vi "数字量输出配置.vi"() -> ()   [LabVIEW 2010] (continued)
              n3559 = local write "单选_第72路"(w107) -> ()
              n3560 = local write "单选_第73路"(w107) -> ()
              n3561 = local write "单选_第74路"(w107) -> ()
              n3562 = local write "单选_第75路"(w107) -> ()
              n3563 = local write "单选_第76路"(w107) -> ()
              n3564 = local write "单选_第77路"(w107) -> ()
              n3565 = local write "单选_第78路"(w107) -> ()
              n3566 = local write "单选_第80路"(w107) -> ()
            }
            frame 40 {
              w108 = TRUE
              w109 = FALSE ("单选_第41路")
              n3567 = local write "单选_第1路"(w108) -> ()
              n3568 = local write "单选_第2路"(w108) -> ()
              n3569 = local write "单选_第3路"(w108) -> ()
              n3570 = local write "单选_第4路"(w108) -> ()
              n3571 = local write "单选_第5路"(w108) -> ()
              n3572 = local write "单选_第6路"(w108) -> ()
              n3573 = local write "单选_第7路"(w108) -> ()
              n3574 = local write "单选_第8路"(w108) -> ()
              n3575 = local write "单选_第9路"(w108) -> ()
              n3576 = local write "单选_第10路"(w108) -> ()
              n3577 = local write "单选_第11路"(w108) -> ()
              n3578 = local write "单选_第12路"(w108) -> ()
              n3579 = local write "单选_第13路"(w108) -> ()
              n3580 = local write "单选_第14路"(w108) -> ()
              n3581 = local write "单选_第15路"(w108) -> ()
              n3582 = local write "单选_第16路"(w108) -> ()
              n3583 = local write "单选_第17路"(w108) -> ()
              n3584 = local write "单选_第18路"(w108) -> ()
              n3585 = local write "单选_第19路"(w108) -> ()
              n3586 = local write "单选_第20路"(w108) -> ()
              n3587 = local write "单选_第21路"(w108) -> ()
              n3588 = local write "单选_第22路"(w108) -> ()
              n3589 = local write "单选_第23路"(w108) -> ()
              n3590 = local write "单选_第24路"(w108) -> ()
              n3591 = local write "单选_第25路"(w108) -> ()
              n3592 = local write "单选_第26路"(w108) -> ()
              n3593 = local write "单选_第27路"(w108) -> ()
              n3594 = local write "单选_第28路"(w108) -> ()
              n3595 = local write "单选_第29路"(w108) -> ()
              n3596 = local write "单选_第30路"(w108) -> ()
              n3597 = local write "单选_第31路"(w108) -> ()
              n3598 = local write "单选_第32路"(w108) -> ()
              n3599 = local write "单选_第33路"(w108) -> ()
              n3600 = local write "单选_第34路"(w108) -> ()
              n3601 = local write "单选_第35路"(w108) -> ()
              n3602 = local write "单选_第36路"(w108) -> ()
              n3603 = local write "单选_第37路"(w108) -> ()
              n3604 = local write "单选_第38路"(w108) -> ()
              n3605 = local write "单选_第39路"(w108) -> ()
              n3606 = local write "单选_第40路"(w108) -> ()
              n3607 = local write "单选_第41路"(w109) -> ()
              n3608 = local write "单选_第42路"(w109) -> ()
              n3609 = local write "单选_第43路"(w109) -> ()
              n3610 = local write "单选_第44路"(w109) -> ()
              n3611 = local write "单选_第45路"(w109) -> ()
              n3612 = local write "单选_第46路"(w109) -> ()
              n3613 = local write "单选_第47路"(w109) -> ()
              n3614 = local write "单选_第48路"(w109) -> ()
              n3615 = local write "单选_第49路"(w109) -> ()
              n3616 = local write "单选_第50路"(w109) -> ()
              n3617 = local write "单选_第51路"(w109) -> ()
              n3618 = local write "单选_第52路"(w109) -> ()
              n3619 = local write "单选_第53路"(w109) -> ()
              n3620 = local write "单选_第54路"(w109) -> ()
              n3621 = local write "单选_第55路"(w109) -> ()
              n3622 = local write "单选_第56路"(w109) -> ()
              n3623 = local write "单选_第57路"(w109) -> ()
              n3624 = local write "单选_第58路"(w109) -> ()
              n3625 = local write "单选_第59路"(w109) -> ()
              n3626 = local write "单选_第60路"(w109) -> ()
              n3627 = local write "单选_第61路"(w109) -> ()
              n3628 = local write "单选_第62路"(w109) -> ()
              n3629 = local write "单选_第63路"(w109) -> ()
              n3630 = local write "单选_第64路"(w109) -> ()
              n3631 = local write "单选_第71路"(w109) -> ()
              n3632 = local write "单选_第79路"(w109) -> ()
              n3633 = local write "单选_第65路"(w109) -> ()
              n3634 = local write "单选_第66路"(w109) -> ()
              n3635 = local write "单选_第67路"(w109) -> ()
              n3636 = local write "单选_第68路"(w109) -> ()
              n3637 = local write "单选_第69路"(w109) -> ()
              n3638 = local write "单选_第70路"(w109) -> ()
              n3639 = local write "单选_第72路"(w109) -> ()
              n3640 = local write "单选_第73路"(w109) -> ()
              n3641 = local write "单选_第74路"(w109) -> ()
              n3642 = local write "单选_第75路"(w109) -> ()
              n3643 = local write "单选_第76路"(w109) -> ()
              n3644 = local write "单选_第77路"(w109) -> ()
              n3645 = local write "单选_第78路"(w109) -> ()
              n3646 = local write "单选_第80路"(w109) -> ()
            }
            frame 41 {
              w110 = TRUE
              w111 = FALSE ("单选_第41路")
              n3647 = local write "单选_第1路"(w110) -> ()
              n3648 = local write "单选_第2路"(w110) -> ()
              n3649 = local write "单选_第3路"(w110) -> ()
              n3650 = local write "单选_第4路"(w110) -> ()
              n3651 = local write "单选_第5路"(w110) -> ()
              n3652 = local write "单选_第6路"(w110) -> ()
              n3653 = local write "单选_第7路"(w110) -> ()
              n3654 = local write "单选_第8路"(w110) -> ()
              n3655 = local write "单选_第9路"(w110) -> ()
              n3656 = local write "单选_第10路"(w110) -> ()
              n3657 = local write "单选_第11路"(w110) -> ()
              n3658 = local write "单选_第12路"(w110) -> ()
              n3659 = local write "单选_第13路"(w110) -> ()
              n3660 = local write "单选_第14路"(w110) -> ()
              n3661 = local write "单选_第15路"(w110) -> ()
              n3662 = local write "单选_第16路"(w110) -> ()
              n3663 = local write "单选_第17路"(w110) -> ()
              n3664 = local write "单选_第18路"(w110) -> ()
              n3665 = local write "单选_第19路"(w110) -> ()
              n3666 = local write "单选_第20路"(w110) -> ()
              n3667 = local write "单选_第21路"(w110) -> ()
              n3668 = local write "单选_第22路"(w110) -> ()
              n3669 = local write "单选_第23路"(w110) -> ()
              n3670 = local write "单选_第24路"(w110) -> ()
              n3671 = local write "单选_第25路"(w110) -> ()
              n3672 = local write "单选_第26路"(w110) -> ()
              n3673 = local write "单选_第27路"(w110) -> ()
              n3674 = local write "单选_第28路"(w110) -> ()
              n3675 = local write "单选_第29路"(w110) -> ()
              n3676 = local write "单选_第30路"(w110) -> ()
              n3677 = local write "单选_第31路"(w110) -> ()
              n3678 = local write "单选_第32路"(w110) -> ()
              n3679 = local write "单选_第33路"(w110) -> ()
              n3680 = local write "单选_第34路"(w110) -> ()
              n3681 = local write "单选_第35路"(w110) -> ()
              n3682 = local write "单选_第36路"(w110) -> ()
              n3683 = local write "单选_第37路"(w110) -> ()
              n3684 = local write "单选_第38路"(w110) -> ()
              n3685 = local write "单选_第39路"(w110) -> ()
              n3686 = local write "单选_第40路"(w110) -> ()
              n3687 = local write "单选_第41路"(w110) -> ()
              n3688 = local write "单选_第42路"(w111) -> ()
              n3689 = local write "单选_第43路"(w111) -> ()
              n3690 = local write "单选_第44路"(w111) -> ()
              n3691 = local write "单选_第45路"(w111) -> ()
              n3692 = local write "单选_第46路"(w111) -> ()
              n3693 = local write "单选_第47路"(w111) -> ()
              n3694 = local write "单选_第48路"(w111) -> ()
              n3695 = local write "单选_第49路"(w111) -> ()
              n3696 = local write "单选_第50路"(w111) -> ()
              n3697 = local write "单选_第51路"(w111) -> ()
              n3698 = local write "单选_第52路"(w111) -> ()
              n3699 = local write "单选_第53路"(w111) -> ()
              n3700 = local write "单选_第54路"(w111) -> ()
              n3701 = local write "单选_第55路"(w111) -> ()
              n3702 = local write "单选_第56路"(w111) -> ()
              n3703 = local write "单选_第57路"(w111) -> ()
              n3704 = local write "单选_第58路"(w111) -> ()
              n3705 = local write "单选_第59路"(w111) -> ()
              n3706 = local write "单选_第60路"(w111) -> ()
              n3707 = local write "单选_第61路"(w111) -> ()
              n3708 = local write "单选_第62路"(w111) -> ()
              n3709 = local write "单选_第63路"(w111) -> ()
              n3710 = local write "单选_第64路"(w111) -> ()
              n3711 = local write "单选_第71路"(w111) -> ()
              n3712 = local write "单选_第79路"(w111) -> ()
              n3713 = local write "单选_第65路"(w111) -> ()
              n3714 = local write "单选_第66路"(w111) -> ()
              n3715 = local write "单选_第67路"(w111) -> ()
              n3716 = local write "单选_第68路"(w111) -> ()
              n3717 = local write "单选_第69路"(w111) -> ()
              n3718 = local write "单选_第70路"(w111) -> ()
              n3719 = local write "单选_第72路"(w111) -> ()
              n3720 = local write "单选_第73路"(w111) -> ()
              n3721 = local write "单选_第74路"(w111) -> ()
              n3722 = local write "单选_第75路"(w111) -> ()
              n3723 = local write "单选_第76路"(w111) -> ()
              n3724 = local write "单选_第77路"(w111) -> ()
              n3725 = local write "单选_第78路"(w111) -> ()
              n3726 = local write "单选_第80路"(w111) -> ()
            }
            frame 42 {
              w112 = TRUE
              w113 = FALSE ("单选_第41路")
              n3727 = local write "单选_第1路"(w112) -> ()
              n3728 = local write "单选_第2路"(w112) -> ()
              n3729 = local write "单选_第3路"(w112) -> ()
              n3730 = local write "单选_第4路"(w112) -> ()
              n3731 = local write "单选_第5路"(w112) -> ()
              n3732 = local write "单选_第6路"(w112) -> ()
              n3733 = local write "单选_第7路"(w112) -> ()
              n3734 = local write "单选_第8路"(w112) -> ()
              n3735 = local write "单选_第9路"(w112) -> ()
              n3736 = local write "单选_第10路"(w112) -> ()
              n3737 = local write "单选_第11路"(w112) -> ()
              n3738 = local write "单选_第12路"(w112) -> ()
              n3739 = local write "单选_第13路"(w112) -> ()
              n3740 = local write "单选_第14路"(w112) -> ()
              n3741 = local write "单选_第15路"(w112) -> ()
              n3742 = local write "单选_第16路"(w112) -> ()
              n3743 = local write "单选_第17路"(w112) -> ()
              n3744 = local write "单选_第18路"(w112) -> ()
              n3745 = local write "单选_第19路"(w112) -> ()
              n3746 = local write "单选_第20路"(w112) -> ()
              n3747 = local write "单选_第21路"(w112) -> ()
              n3748 = local write "单选_第22路"(w112) -> ()
              n3749 = local write "单选_第23路"(w112) -> ()
              n3750 = local write "单选_第24路"(w112) -> ()
              n3751 = local write "单选_第25路"(w112) -> ()
              n3752 = local write "单选_第26路"(w112) -> ()
              n3753 = local write "单选_第27路"(w112) -> ()
              n3754 = local write "单选_第28路"(w112) -> ()
              n3755 = local write "单选_第29路"(w112) -> ()
              n3756 = local write "单选_第30路"(w112) -> ()
              n3757 = local write "单选_第31路"(w112) -> ()
              n3758 = local write "单选_第32路"(w112) -> ()
              n3759 = local write "单选_第33路"(w112) -> ()
              n3760 = local write "单选_第34路"(w112) -> ()
              n3761 = local write "单选_第35路"(w112) -> ()
              n3762 = local write "单选_第36路"(w112) -> ()
              n3763 = local write "单选_第37路"(w112) -> ()
              n3764 = local write "单选_第38路"(w112) -> ()
              n3765 = local write "单选_第39路"(w112) -> ()
              n3766 = local write "单选_第40路"(w112) -> ()
              n3767 = local write "单选_第41路"(w112) -> ()
              n3768 = local write "单选_第42路"(w112) -> ()
              n3769 = local write "单选_第43路"(w113) -> ()
              n3770 = local write "单选_第44路"(w113) -> ()
              n3771 = local write "单选_第45路"(w113) -> ()
              n3772 = local write "单选_第46路"(w113) -> ()
              n3773 = local write "单选_第47路"(w113) -> ()
              n3774 = local write "单选_第48路"(w113) -> ()
              n3775 = local write "单选_第49路"(w113) -> ()
              n3776 = local write "单选_第50路"(w113) -> ()
              n3777 = local write "单选_第51路"(w113) -> ()
              n3778 = local write "单选_第52路"(w113) -> ()
              n3779 = local write "单选_第53路"(w113) -> ()
              n3780 = local write "单选_第54路"(w113) -> ()
              n3781 = local write "单选_第55路"(w113) -> ()
              n3782 = local write "单选_第56路"(w113) -> ()
              n3783 = local write "单选_第57路"(w113) -> ()
              n3784 = local write "单选_第58路"(w113) -> ()
              n3785 = local write "单选_第59路"(w113) -> ()
              n3786 = local write "单选_第60路"(w113) -> ()
              n3787 = local write "单选_第61路"(w113) -> ()
              n3788 = local write "单选_第62路"(w113) -> ()
              n3789 = local write "单选_第63路"(w113) -> ()
              n3790 = local write "单选_第64路"(w113) -> ()
              n3791 = local write "单选_第71路"(w113) -> ()
              n3792 = local write "单选_第79路"(w113) -> ()
              n3793 = local write "单选_第65路"(w113) -> ()
              n3794 = local write "单选_第66路"(w113) -> ()
              n3795 = local write "单选_第67路"(w113) -> ()
              n3796 = local write "单选_第68路"(w113) -> ()
              n3797 = local write "单选_第69路"(w113) -> ()
              n3798 = local write "单选_第70路"(w113) -> ()
              n3799 = local write "单选_第72路"(w113) -> ()
              n3800 = local write "单选_第73路"(w113) -> ()
              n3801 = local write "单选_第74路"(w113) -> ()
              n3802 = local write "单选_第75路"(w113) -> ()
              n3803 = local write "单选_第76路"(w113) -> ()
              n3804 = local write "单选_第77路"(w113) -> ()
              n3805 = local write "单选_第78路"(w113) -> ()
              n3806 = local write "单选_第80路"(w113) -> ()
            }
            frame 43 {
              w114 = TRUE
              w115 = FALSE ("单选_第41路")
              n3807 = local write "单选_第1路"(w114) -> ()
              n3808 = local write "单选_第2路"(w114) -> ()
              n3809 = local write "单选_第3路"(w114) -> ()
              n3810 = local write "单选_第4路"(w114) -> ()
              n3811 = local write "单选_第5路"(w114) -> ()
              n3812 = local write "单选_第6路"(w114) -> ()
              n3813 = local write "单选_第7路"(w114) -> ()
              n3814 = local write "单选_第8路"(w114) -> ()
              n3815 = local write "单选_第9路"(w114) -> ()
              n3816 = local write "单选_第10路"(w114) -> ()
              n3817 = local write "单选_第11路"(w114) -> ()
              n3818 = local write "单选_第12路"(w114) -> ()
              n3819 = local write "单选_第13路"(w114) -> ()
              n3820 = local write "单选_第14路"(w114) -> ()
              n3821 = local write "单选_第15路"(w114) -> ()
              n3822 = local write "单选_第16路"(w114) -> ()
              n3823 = local write "单选_第17路"(w114) -> ()
              n3824 = local write "单选_第18路"(w114) -> ()
              n3825 = local write "单选_第19路"(w114) -> ()
              n3826 = local write "单选_第20路"(w114) -> ()
              n3827 = local write "单选_第21路"(w114) -> ()
              n3828 = local write "单选_第22路"(w114) -> ()
              n3829 = local write "单选_第23路"(w114) -> ()
              n3830 = local write "单选_第24路"(w114) -> ()
              n3831 = local write "单选_第25路"(w114) -> ()
              n3832 = local write "单选_第26路"(w114) -> ()
              n3833 = local write "单选_第27路"(w114) -> ()
              n3834 = local write "单选_第28路"(w114) -> ()
              n3835 = local write "单选_第29路"(w114) -> ()
              n3836 = local write "单选_第30路"(w114) -> ()
              n3837 = local write "单选_第31路"(w114) -> ()
              n3838 = local write "单选_第32路"(w114) -> ()
              n3839 = local write "单选_第33路"(w114) -> ()
              n3840 = local write "单选_第34路"(w114) -> ()
              n3841 = local write "单选_第35路"(w114) -> ()
              n3842 = local write "单选_第36路"(w114) -> ()
              n3843 = local write "单选_第37路"(w114) -> ()
              n3844 = local write "单选_第38路"(w114) -> ()
              n3845 = local write "单选_第39路"(w114) -> ()
              n3846 = local write "单选_第40路"(w114) -> ()
              n3847 = local write "单选_第41路"(w114) -> ()
              n3848 = local write "单选_第42路"(w114) -> ()
              n3849 = local write "单选_第43路"(w114) -> ()
              n3850 = local write "单选_第44路"(w115) -> ()
              n3851 = local write "单选_第45路"(w115) -> ()
              n3852 = local write "单选_第46路"(w115) -> ()
              n3853 = local write "单选_第47路"(w115) -> ()
              n3854 = local write "单选_第48路"(w115) -> ()
              n3855 = local write "单选_第49路"(w115) -> ()
              n3856 = local write "单选_第50路"(w115) -> ()
              n3857 = local write "单选_第51路"(w115) -> ()
              n3858 = local write "单选_第52路"(w115) -> ()
              n3859 = local write "单选_第53路"(w115) -> ()
              n3860 = local write "单选_第54路"(w115) -> ()
              n3861 = local write "单选_第55路"(w115) -> ()
              n3862 = local write "单选_第56路"(w115) -> ()
              n3863 = local write "单选_第57路"(w115) -> ()
              n3864 = local write "单选_第58路"(w115) -> ()
              n3865 = local write "单选_第59路"(w115) -> ()
              n3866 = local write "单选_第60路"(w115) -> ()
              n3867 = local write "单选_第61路"(w115) -> ()
              n3868 = local write "单选_第62路"(w115) -> ()
              n3869 = local write "单选_第63路"(w115) -> ()
              n3870 = local write "单选_第64路"(w115) -> ()
              n3871 = local write "单选_第71路"(w115) -> ()
              n3872 = local write "单选_第79路"(w115) -> ()
              n3873 = local write "单选_第65路"(w115) -> ()
              n3874 = local write "单选_第66路"(w115) -> ()
              n3875 = local write "单选_第67路"(w115) -> ()
              n3876 = local write "单选_第68路"(w115) -> ()
              n3877 = local write "单选_第69路"(w115) -> ()
              n3878 = local write "单选_第70路"(w115) -> ()
              n3879 = local write "单选_第72路"(w115) -> ()
              n3880 = local write "单选_第73路"(w115) -> ()
              n3881 = local write "单选_第74路"(w115) -> ()
              n3882 = local write "单选_第75路"(w115) -> ()
              n3883 = local write "单选_第76路"(w115) -> ()
              n3884 = local write "单选_第77路"(w115) -> ()
              n3885 = local write "单选_第78路"(w115) -> ()
              n3886 = local write "单选_第80路"(w115) -> ()
            }
            frame 44 {
              w116 = TRUE
              w117 = FALSE ("单选_第41路")
              n3887 = local write "单选_第1路"(w116) -> ()
              n3888 = local write "单选_第2路"(w116) -> ()
              n3889 = local write "单选_第3路"(w116) -> ()
              n3890 = local write "单选_第4路"(w116) -> ()
              n3891 = local write "单选_第5路"(w116) -> ()
              n3892 = local write "单选_第6路"(w116) -> ()
              n3893 = local write "单选_第7路"(w116) -> ()
              n3894 = local write "单选_第8路"(w116) -> ()
              n3895 = local write "单选_第9路"(w116) -> ()
              n3896 = local write "单选_第10路"(w116) -> ()
              n3897 = local write "单选_第11路"(w116) -> ()
              n3898 = local write "单选_第12路"(w116) -> ()
              n3899 = local write "单选_第13路"(w116) -> ()
              n3900 = local write "单选_第14路"(w116) -> ()
              n3901 = local write "单选_第15路"(w116) -> ()
              n3902 = local write "单选_第16路"(w116) -> ()
              n3903 = local write "单选_第17路"(w116) -> ()
              n3904 = local write "单选_第18路"(w116) -> ()
              n3905 = local write "单选_第19路"(w116) -> ()
              n3906 = local write "单选_第20路"(w116) -> ()
              n3907 = local write "单选_第21路"(w116) -> ()
              n3908 = local write "单选_第22路"(w116) -> ()
              n3909 = local write "单选_第23路"(w116) -> ()
              n3910 = local write "单选_第24路"(w116) -> ()
              n3911 = local write "单选_第25路"(w116) -> ()
              n3912 = local write "单选_第26路"(w116) -> ()
              n3913 = local write "单选_第27路"(w116) -> ()
              n3914 = local write "单选_第28路"(w116) -> ()
              n3915 = local write "单选_第29路"(w116) -> ()
              n3916 = local write "单选_第30路"(w116) -> ()
              n3917 = local write "单选_第31路"(w116) -> ()
              n3918 = local write "单选_第32路"(w116) -> ()
              n3919 = local write "单选_第33路"(w116) -> ()
              n3920 = local write "单选_第34路"(w116) -> ()
              n3921 = local write "单选_第35路"(w116) -> ()
              n3922 = local write "单选_第36路"(w116) -> ()
              n3923 = local write "单选_第37路"(w116) -> ()
              n3924 = local write "单选_第38路"(w116) -> ()
              n3925 = local write "单选_第39路"(w116) -> ()
              n3926 = local write "单选_第40路"(w116) -> ()
              n3927 = local write "单选_第41路"(w116) -> ()
              n3928 = local write "单选_第42路"(w116) -> ()
              n3929 = local write "单选_第43路"(w116) -> ()
              n3930 = local write "单选_第44路"(w116) -> ()
              n3931 = local write "单选_第45路"(w117) -> ()
              n3932 = local write "单选_第46路"(w117) -> ()
              n3933 = local write "单选_第47路"(w117) -> ()
              n3934 = local write "单选_第48路"(w117) -> ()
              n3935 = local write "单选_第49路"(w117) -> ()
              n3936 = local write "单选_第50路"(w117) -> ()
              n3937 = local write "单选_第51路"(w117) -> ()
              n3938 = local write "单选_第52路"(w117) -> ()
              n3939 = local write "单选_第53路"(w117) -> ()
              n3940 = local write "单选_第54路"(w117) -> ()
              n3941 = local write "单选_第55路"(w117) -> ()
              n3942 = local write "单选_第56路"(w117) -> ()
              n3943 = local write "单选_第57路"(w117) -> ()
              n3944 = local write "单选_第58路"(w117) -> ()
              n3945 = local write "单选_第59路"(w117) -> ()
              n3946 = local write "单选_第60路"(w117) -> ()
              n3947 = local write "单选_第61路"(w117) -> ()
              n3948 = local write "单选_第62路"(w117) -> ()
              n3949 = local write "单选_第63路"(w117) -> ()
              n3950 = local write "单选_第64路"(w117) -> ()
              n3951 = local write "单选_第71路"(w117) -> ()
              n3952 = local write "单选_第79路"(w117) -> ()
              n3953 = local write "单选_第65路"(w117) -> ()
              n3954 = local write "单选_第66路"(w117) -> ()
              n3955 = local write "单选_第67路"(w117) -> ()
              n3956 = local write "单选_第68路"(w117) -> ()
              n3957 = local write "单选_第69路"(w117) -> ()
              n3958 = local write "单选_第70路"(w117) -> ()
              n3959 = local write "单选_第72路"(w117) -> ()
              n3960 = local write "单选_第73路"(w117) -> ()
              n3961 = local write "单选_第74路"(w117) -> ()
              n3962 = local write "单选_第75路"(w117) -> ()
              n3963 = local write "单选_第76路"(w117) -> ()
              n3964 = local write "单选_第77路"(w117) -> ()
              n3965 = local write "单选_第78路"(w117) -> ()
              n3966 = local write "单选_第80路"(w117) -> ()
            }
            frame 45 {
              w118 = TRUE
              w119 = FALSE ("单选_第41路")
              n3967 = local write "单选_第1路"(w118) -> ()
              n3968 = local write "单选_第2路"(w118) -> ()
              n3969 = local write "单选_第3路"(w118) -> ()
              n3970 = local write "单选_第4路"(w118) -> ()
              n3971 = local write "单选_第5路"(w118) -> ()
              n3972 = local write "单选_第6路"(w118) -> ()
              n3973 = local write "单选_第7路"(w118) -> ()
              n3974 = local write "单选_第8路"(w118) -> ()
              n3975 = local write "单选_第9路"(w118) -> ()
              n3976 = local write "单选_第10路"(w118) -> ()
              n3977 = local write "单选_第11路"(w118) -> ()
              n3978 = local write "单选_第12路"(w118) -> ()
              n3979 = local write "单选_第13路"(w118) -> ()
              n3980 = local write "单选_第14路"(w118) -> ()
              n3981 = local write "单选_第15路"(w118) -> ()
              n3982 = local write "单选_第16路"(w118) -> ()
              n3983 = local write "单选_第17路"(w118) -> ()
              n3984 = local write "单选_第18路"(w118) -> ()
              n3985 = local write "单选_第19路"(w118) -> ()
              n3986 = local write "单选_第20路"(w118) -> ()
              n3987 = local write "单选_第21路"(w118) -> ()
              n3988 = local write "单选_第22路"(w118) -> ()
              n3989 = local write "单选_第23路"(w118) -> ()
              n3990 = local write "单选_第24路"(w118) -> ()
              n3991 = local write "单选_第25路"(w118) -> ()
              n3992 = local write "单选_第26路"(w118) -> ()
              n3993 = local write "单选_第27路"(w118) -> ()
              n3994 = local write "单选_第28路"(w118) -> ()
              n3995 = local write "单选_第29路"(w118) -> ()
              n3996 = local write "单选_第30路"(w118) -> ()
              n3997 = local write "单选_第31路"(w118) -> ()
              n3998 = local write "单选_第32路"(w118) -> ()
              n3999 = local write "单选_第33路"(w118) -> ()
              n4000 = local write "单选_第34路"(w118) -> ()
              n4001 = local write "单选_第35路"(w118) -> ()
              n4002 = local write "单选_第36路"(w118) -> ()
              n4003 = local write "单选_第37路"(w118) -> ()
              n4004 = local write "单选_第38路"(w118) -> ()
              n4005 = local write "单选_第39路"(w118) -> ()
              n4006 = local write "单选_第40路"(w118) -> ()
              n4007 = local write "单选_第41路"(w118) -> ()
              n4008 = local write "单选_第42路"(w118) -> ()
              n4009 = local write "单选_第43路"(w118) -> ()
              n4010 = local write "单选_第44路"(w118) -> ()
              n4011 = local write "单选_第45路"(w118) -> ()
              n4012 = local write "单选_第46路"(w119) -> ()
              n4013 = local write "单选_第47路"(w119) -> ()
              n4014 = local write "单选_第48路"(w119) -> ()
              n4015 = local write "单选_第49路"(w119) -> ()
              n4016 = local write "单选_第50路"(w119) -> ()
              n4017 = local write "单选_第51路"(w119) -> ()
              n4018 = local write "单选_第52路"(w119) -> ()
              n4019 = local write "单选_第53路"(w119) -> ()
              n4020 = local write "单选_第54路"(w119) -> ()
              n4021 = local write "单选_第55路"(w119) -> ()
              n4022 = local write "单选_第56路"(w119) -> ()
              n4023 = local write "单选_第57路"(w119) -> ()
              n4024 = local write "单选_第58路"(w119) -> ()
              n4025 = local write "单选_第59路"(w119) -> ()
              n4026 = local write "单选_第60路"(w119) -> ()
              n4027 = local write "单选_第61路"(w119) -> ()
              n4028 = local write "单选_第62路"(w119) -> ()
              n4029 = local write "单选_第63路"(w119) -> ()
              n4030 = local write "单选_第64路"(w119) -> ()
              n4031 = local write "单选_第71路"(w119) -> ()
              n4032 = local write "单选_第79路"(w119) -> ()
              n4033 = local write "单选_第65路"(w119) -> ()
              n4034 = local write "单选_第66路"(w119) -> ()
              n4035 = local write "单选_第67路"(w119) -> ()
              n4036 = local write "单选_第68路"(w119) -> ()
              n4037 = local write "单选_第69路"(w119) -> ()
              n4038 = local write "单选_第70路"(w119) -> ()
              n4039 = local write "单选_第72路"(w119) -> ()
              n4040 = local write "单选_第73路"(w119) -> ()
              n4041 = local write "单选_第74路"(w119) -> ()
              n4042 = local write "单选_第75路"(w119) -> ()
              n4043 = local write "单选_第76路"(w119) -> ()
              n4044 = local write "单选_第77路"(w119) -> ()
              n4045 = local write "单选_第78路"(w119) -> ()
              n4046 = local write "单选_第80路"(w119) -> ()
            }
            frame 46 {
              w120 = TRUE
              w121 = FALSE ("单选_第41路")
              n4047 = local write "单选_第1路"(w120) -> ()
              n4048 = local write "单选_第2路"(w120) -> ()
              n4049 = local write "单选_第3路"(w120) -> ()
              n4050 = local write "单选_第4路"(w120) -> ()
              n4051 = local write "单选_第5路"(w120) -> ()
              n4052 = local write "单选_第6路"(w120) -> ()
              n4053 = local write "单选_第7路"(w120) -> ()
              n4054 = local write "单选_第8路"(w120) -> ()
              n4055 = local write "单选_第9路"(w120) -> ()
              n4056 = local write "单选_第10路"(w120) -> ()
              n4057 = local write "单选_第11路"(w120) -> ()
              n4058 = local write "单选_第12路"(w120) -> ()
              n4059 = local write "单选_第13路"(w120) -> ()
              n4060 = local write "单选_第14路"(w120) -> ()
              n4061 = local write "单选_第15路"(w120) -> ()
              n4062 = local write "单选_第16路"(w120) -> ()
              n4063 = local write "单选_第17路"(w120) -> ()
              n4064 = local write "单选_第18路"(w120) -> ()
              n4065 = local write "单选_第19路"(w120) -> ()
              n4066 = local write "单选_第20路"(w120) -> ()
              n4067 = local write "单选_第21路"(w120) -> ()
              n4068 = local write "单选_第22路"(w120) -> ()
              n4069 = local write "单选_第23路"(w120) -> ()
              n4070 = local write "单选_第24路"(w120) -> ()
              n4071 = local write "单选_第25路"(w120) -> ()
              n4072 = local write "单选_第26路"(w120) -> ()
              n4073 = local write "单选_第27路"(w120) -> ()
              n4074 = local write "单选_第28路"(w120) -> ()
              n4075 = local write "单选_第29路"(w120) -> ()
              n4076 = local write "单选_第30路"(w120) -> ()
              n4077 = local write "单选_第31路"(w120) -> ()
              n4078 = local write "单选_第32路"(w120) -> ()
              n4079 = local write "单选_第33路"(w120) -> ()
              n4080 = local write "单选_第34路"(w120) -> ()
              n4081 = local write "单选_第35路"(w120) -> ()
              n4082 = local write "单选_第36路"(w120) -> ()
              n4083 = local write "单选_第37路"(w120) -> ()
              n4084 = local write "单选_第38路"(w120) -> ()
              n4085 = local write "单选_第39路"(w120) -> ()
              n4086 = local write "单选_第40路"(w120) -> ()
              n4087 = local write "单选_第41路"(w120) -> ()
              n4088 = local write "单选_第42路"(w120) -> ()
              n4089 = local write "单选_第43路"(w120) -> ()
              n4090 = local write "单选_第44路"(w120) -> ()
              n4091 = local write "单选_第45路"(w120) -> ()
              n4092 = local write "单选_第46路"(w120) -> ()
              n4093 = local write "单选_第47路"(w121) -> ()
              n4094 = local write "单选_第48路"(w121) -> ()
              n4095 = local write "单选_第49路"(w121) -> ()
              n4096 = local write "单选_第50路"(w121) -> ()
              n4097 = local write "单选_第51路"(w121) -> ()
              n4098 = local write "单选_第52路"(w121) -> ()
              n4099 = local write "单选_第53路"(w121) -> ()
              n4100 = local write "单选_第54路"(w121) -> ()
              n4101 = local write "单选_第55路"(w121) -> ()
              n4102 = local write "单选_第56路"(w121) -> ()
              n4103 = local write "单选_第57路"(w121) -> ()
              n4104 = local write "单选_第58路"(w121) -> ()
              n4105 = local write "单选_第59路"(w121) -> ()
              n4106 = local write "单选_第60路"(w121) -> ()
              n4107 = local write "单选_第61路"(w121) -> ()
              n4108 = local write "单选_第62路"(w121) -> ()
              n4109 = local write "单选_第63路"(w121) -> ()
              n4110 = local write "单选_第64路"(w121) -> ()
              n4111 = local write "单选_第71路"(w121) -> ()
              n4112 = local write "单选_第79路"(w121) -> ()
              n4113 = local write "单选_第65路"(w121) -> ()
              n4114 = local write "单选_第66路"(w121) -> ()
              n4115 = local write "单选_第67路"(w121) -> ()
              n4116 = local write "单选_第68路"(w121) -> ()
              n4117 = local write "单选_第69路"(w121) -> ()
              n4118 = local write "单选_第70路"(w121) -> ()
              n4119 = local write "单选_第72路"(w121) -> ()
              n4120 = local write "单选_第73路"(w121) -> ()
              n4121 = local write "单选_第74路"(w121) -> ()
              n4122 = local write "单选_第75路"(w121) -> ()
              n4123 = local write "单选_第76路"(w121) -> ()
              n4124 = local write "单选_第77路"(w121) -> ()
              n4125 = local write "单选_第78路"(w121) -> ()
              n4126 = local write "单选_第80路"(w121) -> ()
            }
            frame 47 {
              w122 = TRUE
              w123 = FALSE ("单选_第41路")
              n4127 = local write "单选_第1路"(w122) -> ()
              n4128 = local write "单选_第2路"(w122) -> ()
              n4129 = local write "单选_第3路"(w122) -> ()
              n4130 = local write "单选_第4路"(w122) -> ()
              n4131 = local write "单选_第5路"(w122) -> ()
              n4132 = local write "单选_第6路"(w122) -> ()
              n4133 = local write "单选_第7路"(w122) -> ()
              n4134 = local write "单选_第8路"(w122) -> ()
              n4135 = local write "单选_第9路"(w122) -> ()
              n4136 = local write "单选_第10路"(w122) -> ()
              n4137 = local write "单选_第11路"(w122) -> ()
              n4138 = local write "单选_第12路"(w122) -> ()
              n4139 = local write "单选_第13路"(w122) -> ()
              n4140 = local write "单选_第14路"(w122) -> ()
              n4141 = local write "单选_第15路"(w122) -> ()
              n4142 = local write "单选_第16路"(w122) -> ()
              n4143 = local write "单选_第17路"(w122) -> ()
              n4144 = local write "单选_第18路"(w122) -> ()
              n4145 = local write "单选_第19路"(w122) -> ()
              n4146 = local write "单选_第20路"(w122) -> ()
              n4147 = local write "单选_第21路"(w122) -> ()
              n4148 = local write "单选_第22路"(w122) -> ()
              n4149 = local write "单选_第23路"(w122) -> ()
              n4150 = local write "单选_第24路"(w122) -> ()
              n4151 = local write "单选_第25路"(w122) -> ()
              n4152 = local write "单选_第26路"(w122) -> ()
              n4153 = local write "单选_第27路"(w122) -> ()
              n4154 = local write "单选_第28路"(w122) -> ()
              n4155 = local write "单选_第29路"(w122) -> ()
              n4156 = local write "单选_第30路"(w122) -> ()
              n4157 = local write "单选_第31路"(w122) -> ()
              n4158 = local write "单选_第32路"(w122) -> ()
              n4159 = local write "单选_第33路"(w122) -> ()
              n4160 = local write "单选_第34路"(w122) -> ()
              n4161 = local write "单选_第35路"(w122) -> ()
              n4162 = local write "单选_第36路"(w122) -> ()
              n4163 = local write "单选_第37路"(w122) -> ()
              n4164 = local write "单选_第38路"(w122) -> ()
              n4165 = local write "单选_第39路"(w122) -> ()
              n4166 = local write "单选_第40路"(w122) -> ()
              n4167 = local write "单选_第41路"(w122) -> ()
              n4168 = local write "单选_第42路"(w122) -> ()
              n4169 = local write "单选_第43路"(w122) -> ()
              n4170 = local write "单选_第44路"(w122) -> ()
              n4171 = local write "单选_第45路"(w122) -> ()
              n4172 = local write "单选_第46路"(w122) -> ()
              n4173 = local write "单选_第47路"(w122) -> ()
              n4174 = local write "单选_第48路"(w123) -> ()
              n4175 = local write "单选_第49路"(w123) -> ()
              n4176 = local write "单选_第50路"(w123) -> ()
              n4177 = local write "单选_第51路"(w123) -> ()
              n4178 = local write "单选_第52路"(w123) -> ()
              n4179 = local write "单选_第53路"(w123) -> ()
              n4180 = local write "单选_第54路"(w123) -> ()
              n4181 = local write "单选_第55路"(w123) -> ()
              n4182 = local write "单选_第56路"(w123) -> ()
              n4183 = local write "单选_第57路"(w123) -> ()
              n4184 = local write "单选_第58路"(w123) -> ()
              n4185 = local write "单选_第59路"(w123) -> ()
              n4186 = local write "单选_第60路"(w123) -> ()
              n4187 = local write "单选_第61路"(w123) -> ()
              n4188 = local write "单选_第62路"(w123) -> ()
              n4189 = local write "单选_第63路"(w123) -> ()
              n4190 = local write "单选_第64路"(w123) -> ()
              n4191 = local write "单选_第71路"(w123) -> ()
              n4192 = local write "单选_第79路"(w123) -> ()
              n4193 = local write "单选_第65路"(w123) -> ()
              n4194 = local write "单选_第66路"(w123) -> ()
              n4195 = local write "单选_第67路"(w123) -> ()
              n4196 = local write "单选_第68路"(w123) -> ()
              n4197 = local write "单选_第69路"(w123) -> ()
              n4198 = local write "单选_第70路"(w123) -> ()
              n4199 = local write "单选_第72路"(w123) -> ()
              n4200 = local write "单选_第73路"(w123) -> ()
              n4201 = local write "单选_第74路"(w123) -> ()
              n4202 = local write "单选_第75路"(w123) -> ()
              n4203 = local write "单选_第76路"(w123) -> ()
              n4204 = local write "单选_第77路"(w123) -> ()
              n4205 = local write "单选_第78路"(w123) -> ()
              n4206 = local write "单选_第80路"(w123) -> ()
            }
            frame 48 {
              w124 = TRUE
              w125 = FALSE ("单选_第41路")
              n4207 = local write "单选_第1路"(w124) -> ()
              n4208 = local write "单选_第2路"(w124) -> ()
              n4209 = local write "单选_第3路"(w124) -> ()
              n4210 = local write "单选_第4路"(w124) -> ()
              n4211 = local write "单选_第5路"(w124) -> ()
              n4212 = local write "单选_第6路"(w124) -> ()
              n4213 = local write "单选_第7路"(w124) -> ()
              n4214 = local write "单选_第8路"(w124) -> ()
              n4215 = local write "单选_第9路"(w124) -> ()
              n4216 = local write "单选_第10路"(w124) -> ()
              n4217 = local write "单选_第11路"(w124) -> ()
              n4218 = local write "单选_第12路"(w124) -> ()
              n4219 = local write "单选_第13路"(w124) -> ()
              n4220 = local write "单选_第14路"(w124) -> ()
              n4221 = local write "单选_第15路"(w124) -> ()
              n4222 = local write "单选_第16路"(w124) -> ()
              n4223 = local write "单选_第17路"(w124) -> ()
              n4224 = local write "单选_第18路"(w124) -> ()
              n4225 = local write "单选_第19路"(w124) -> ()
              n4226 = local write "单选_第20路"(w124) -> ()
              n4227 = local write "单选_第21路"(w124) -> ()
              n4228 = local write "单选_第22路"(w124) -> ()
              n4229 = local write "单选_第23路"(w124) -> ()
              n4230 = local write "单选_第24路"(w124) -> ()
              n4231 = local write "单选_第25路"(w124) -> ()
              n4232 = local write "单选_第26路"(w124) -> ()
              n4233 = local write "单选_第27路"(w124) -> ()
              n4234 = local write "单选_第28路"(w124) -> ()
              n4235 = local write "单选_第29路"(w124) -> ()
              n4236 = local write "单选_第30路"(w124) -> ()
              n4237 = local write "单选_第31路"(w124) -> ()
              n4238 = local write "单选_第32路"(w124) -> ()
              n4239 = local write "单选_第33路"(w124) -> ()
              n4240 = local write "单选_第34路"(w124) -> ()
              n4241 = local write "单选_第35路"(w124) -> ()
              n4242 = local write "单选_第36路"(w124) -> ()
              n4243 = local write "单选_第37路"(w124) -> ()
              n4244 = local write "单选_第38路"(w124) -> ()
              n4245 = local write "单选_第39路"(w124) -> ()
              n4246 = local write "单选_第40路"(w124) -> ()
              n4247 = local write "单选_第41路"(w124) -> ()
              n4248 = local write "单选_第42路"(w124) -> ()
              n4249 = local write "单选_第43路"(w124) -> ()
              n4250 = local write "单选_第44路"(w124) -> ()
              n4251 = local write "单选_第45路"(w124) -> ()
              n4252 = local write "单选_第46路"(w124) -> ()
              n4253 = local write "单选_第47路"(w124) -> ()
              n4254 = local write "单选_第48路"(w124) -> ()
              n4255 = local write "单选_第49路"(w125) -> ()
              n4256 = local write "单选_第50路"(w125) -> ()
              n4257 = local write "单选_第51路"(w125) -> ()
              n4258 = local write "单选_第52路"(w125) -> ()
              n4259 = local write "单选_第53路"(w125) -> ()
              n4260 = local write "单选_第54路"(w125) -> ()
              n4261 = local write "单选_第55路"(w125) -> ()
              n4262 = local write "单选_第56路"(w125) -> ()
              n4263 = local write "单选_第57路"(w125) -> ()
              n4264 = local write "单选_第58路"(w125) -> ()
              n4265 = local write "单选_第59路"(w125) -> ()
              n4266 = local write "单选_第60路"(w125) -> ()
              n4267 = local write "单选_第61路"(w125) -> ()
              n4268 = local write "单选_第62路"(w125) -> ()
              n4269 = local write "单选_第63路"(w125) -> ()
              n4270 = local write "单选_第64路"(w125) -> ()
              n4271 = local write "单选_第71路"(w125) -> ()
              n4272 = local write "单选_第79路"(w125) -> ()
              n4273 = local write "单选_第65路"(w125) -> ()
              n4274 = local write "单选_第66路"(w125) -> ()
              n4275 = local write "单选_第67路"(w125) -> ()
              n4276 = local write "单选_第68路"(w125) -> ()
              n4277 = local write "单选_第69路"(w125) -> ()
              n4278 = local write "单选_第70路"(w125) -> ()
              n4279 = local write "单选_第72路"(w125) -> ()
              n4280 = local write "单选_第73路"(w125) -> ()
              n4281 = local write "单选_第74路"(w125) -> ()
              n4282 = local write "单选_第75路"(w125) -> ()
              n4283 = local write "单选_第76路"(w125) -> ()
              n4284 = local write "单选_第77路"(w125) -> ()
              n4285 = local write "单选_第78路"(w125) -> ()
              n4286 = local write "单选_第80路"(w125) -> ()
            }
            frame 49 {
              w126 = TRUE
              w127 = FALSE ("单选_第41路")
              n4287 = local write "单选_第1路"(w126) -> ()
              n4288 = local write "单选_第2路"(w126) -> ()
              n4289 = local write "单选_第3路"(w126) -> ()
              n4290 = local write "单选_第4路"(w126) -> ()
              n4291 = local write "单选_第5路"(w126) -> ()
              n4292 = local write "单选_第6路"(w126) -> ()
              n4293 = local write "单选_第7路"(w126) -> ()
              n4294 = local write "单选_第8路"(w126) -> ()
              n4295 = local write "单选_第9路"(w126) -> ()
              n4296 = local write "单选_第10路"(w126) -> ()
              n4297 = local write "单选_第11路"(w126) -> ()
              n4298 = local write "单选_第12路"(w126) -> ()
              n4299 = local write "单选_第13路"(w126) -> ()
              n4300 = local write "单选_第14路"(w126) -> ()
              n4301 = local write "单选_第15路"(w126) -> ()
              n4302 = local write "单选_第16路"(w126) -> ()
              n4303 = local write "单选_第17路"(w126) -> ()
              n4304 = local write "单选_第18路"(w126) -> ()
              n4305 = local write "单选_第19路"(w126) -> ()
              n4306 = local write "单选_第20路"(w126) -> ()
              n4307 = local write "单选_第21路"(w126) -> ()
              n4308 = local write "单选_第22路"(w126) -> ()
              n4309 = local write "单选_第23路"(w126) -> ()
              n4310 = local write "单选_第24路"(w126) -> ()
              n4311 = local write "单选_第25路"(w126) -> ()
              n4312 = local write "单选_第26路"(w126) -> ()
              n4313 = local write "单选_第27路"(w126) -> ()
              n4314 = local write "单选_第28路"(w126) -> ()
              n4315 = local write "单选_第29路"(w126) -> ()
              n4316 = local write "单选_第30路"(w126) -> ()
              n4317 = local write "单选_第31路"(w126) -> ()
              n4318 = local write "单选_第32路"(w126) -> ()
              n4319 = local write "单选_第33路"(w126) -> ()
              n4320 = local write "单选_第34路"(w126) -> ()
              n4321 = local write "单选_第35路"(w126) -> ()
              n4322 = local write "单选_第36路"(w126) -> ()
              n4323 = local write "单选_第37路"(w126) -> ()
              n4324 = local write "单选_第38路"(w126) -> ()
              n4325 = local write "单选_第39路"(w126) -> ()
              n4326 = local write "单选_第40路"(w126) -> ()
              n4327 = local write "单选_第41路"(w126) -> ()
              n4328 = local write "单选_第42路"(w126) -> ()
              n4329 = local write "单选_第43路"(w126) -> ()
              n4330 = local write "单选_第44路"(w126) -> ()
              n4331 = local write "单选_第45路"(w126) -> ()
              n4332 = local write "单选_第46路"(w126) -> ()
              n4333 = local write "单选_第47路"(w126) -> ()
              n4334 = local write "单选_第48路"(w126) -> ()
              n4335 = local write "单选_第49路"(w126) -> ()
              n4336 = local write "单选_第50路"(w127) -> ()
              n4337 = local write "单选_第51路"(w127) -> ()
              n4338 = local write "单选_第52路"(w127) -> ()
              n4339 = local write "单选_第53路"(w127) -> ()
              n4340 = local write "单选_第54路"(w127) -> ()
              n4341 = local write "单选_第55路"(w127) -> ()
              n4342 = local write "单选_第56路"(w127) -> ()
              n4343 = local write "单选_第57路"(w127) -> ()
              n4344 = local write "单选_第58路"(w127) -> ()
              n4345 = local write "单选_第59路"(w127) -> ()
              n4346 = local write "单选_第60路"(w127) -> ()
              n4347 = local write "单选_第61路"(w127) -> ()
              n4348 = local write "单选_第62路"(w127) -> ()
              n4349 = local write "单选_第63路"(w127) -> ()
              n4350 = local write "单选_第64路"(w127) -> ()
              n4351 = local write "单选_第71路"(w127) -> ()
              n4352 = local write "单选_第79路"(w127) -> ()
              n4353 = local write "单选_第65路"(w127) -> ()
              n4354 = local write "单选_第66路"(w127) -> ()
              n4355 = local write "单选_第67路"(w127) -> ()
              n4356 = local write "单选_第68路"(w127) -> ()
              n4357 = local write "单选_第69路"(w127) -> ()
              n4358 = local write "单选_第70路"(w127) -> ()
              n4359 = local write "单选_第72路"(w127) -> ()
              n4360 = local write "单选_第73路"(w127) -> ()
              n4361 = local write "单选_第74路"(w127) -> ()
              n4362 = local write "单选_第75路"(w127) -> ()
              n4363 = local write "单选_第76路"(w127) -> ()
              n4364 = local write "单选_第77路"(w127) -> ()
              n4365 = local write "单选_第78路"(w127) -> ()
              n4366 = local write "单选_第80路"(w127) -> ()
            }
            frame 50 {
              w128 = TRUE
              w129 = FALSE ("单选_第41路")
              n4367 = local write "单选_第1路"(w128) -> ()
              n4368 = local write "单选_第2路"(w128) -> ()
              n4369 = local write "单选_第3路"(w128) -> ()
              n4370 = local write "单选_第4路"(w128) -> ()
              n4371 = local write "单选_第5路"(w128) -> ()
              n4372 = local write "单选_第6路"(w128) -> ()
              n4373 = local write "单选_第7路"(w128) -> ()
              n4374 = local write "单选_第8路"(w128) -> ()
              n4375 = local write "单选_第9路"(w128) -> ()
              n4376 = local write "单选_第10路"(w128) -> ()
              n4377 = local write "单选_第11路"(w128) -> ()
              n4378 = local write "单选_第12路"(w128) -> ()
              n4379 = local write "单选_第13路"(w128) -> ()
              n4380 = local write "单选_第14路"(w128) -> ()
              n4381 = local write "单选_第15路"(w128) -> ()
              n4382 = local write "单选_第16路"(w128) -> ()
              n4383 = local write "单选_第17路"(w128) -> ()
              n4384 = local write "单选_第18路"(w128) -> ()
              n4385 = local write "单选_第19路"(w128) -> ()
              n4386 = local write "单选_第20路"(w128) -> ()
              n4387 = local write "单选_第21路"(w128) -> ()
              n4388 = local write "单选_第22路"(w128) -> ()
              n4389 = local write "单选_第23路"(w128) -> ()
              n4390 = local write "单选_第24路"(w128) -> ()
              n4391 = local write "单选_第25路"(w128) -> ()
              n4392 = local write "单选_第26路"(w128) -> ()
              n4393 = local write "单选_第27路"(w128) -> ()
              n4394 = local write "单选_第28路"(w128) -> ()
              n4395 = local write "单选_第29路"(w128) -> ()
              n4396 = local write "单选_第30路"(w128) -> ()
              n4397 = local write "单选_第31路"(w128) -> ()
              n4398 = local write "单选_第32路"(w128) -> ()
              n4399 = local write "单选_第33路"(w128) -> ()
              n4400 = local write "单选_第34路"(w128) -> ()
              n4401 = local write "单选_第35路"(w128) -> ()
              n4402 = local write "单选_第36路"(w128) -> ()
              n4403 = local write "单选_第37路"(w128) -> ()
              n4404 = local write "单选_第38路"(w128) -> ()
              n4405 = local write "单选_第39路"(w128) -> ()
              n4406 = local write "单选_第40路"(w128) -> ()
              n4407 = local write "单选_第41路"(w128) -> ()
              n4408 = local write "单选_第42路"(w128) -> ()
              n4409 = local write "单选_第43路"(w128) -> ()
              n4410 = local write "单选_第44路"(w128) -> ()
              n4411 = local write "单选_第45路"(w128) -> ()
              n4412 = local write "单选_第46路"(w128) -> ()
              n4413 = local write "单选_第47路"(w128) -> ()
              n4414 = local write "单选_第48路"(w128) -> ()
              n4415 = local write "单选_第49路"(w128) -> ()
              n4416 = local write "单选_第50路"(w128) -> ()
              n4417 = local write "单选_第51路"(w129) -> ()
              n4418 = local write "单选_第52路"(w129) -> ()
              n4419 = local write "单选_第53路"(w129) -> ()
              n4420 = local write "单选_第54路"(w129) -> ()
              n4421 = local write "单选_第55路"(w129) -> ()
              n4422 = local write "单选_第56路"(w129) -> ()
              n4423 = local write "单选_第57路"(w129) -> ()
              n4424 = local write "单选_第58路"(w129) -> ()
              n4425 = local write "单选_第59路"(w129) -> ()
              n4426 = local write "单选_第60路"(w129) -> ()
              n4427 = local write "单选_第61路"(w129) -> ()
              n4428 = local write "单选_第62路"(w129) -> ()
              n4429 = local write "单选_第63路"(w129) -> ()
              n4430 = local write "单选_第64路"(w129) -> ()
              n4431 = local write "单选_第71路"(w129) -> ()
              n4432 = local write "单选_第79路"(w129) -> ()
              n4433 = local write "单选_第65路"(w129) -> ()
              n4434 = local write "单选_第66路"(w129) -> ()
              n4435 = local write "单选_第67路"(w129) -> ()
              n4436 = local write "单选_第68路"(w129) -> ()
              n4437 = local write "单选_第69路"(w129) -> ()
              n4438 = local write "单选_第70路"(w129) -> ()
              n4439 = local write "单选_第72路"(w129) -> ()
              n4440 = local write "单选_第73路"(w129) -> ()
              n4441 = local write "单选_第74路"(w129) -> ()
              n4442 = local write "单选_第75路"(w129) -> ()
              n4443 = local write "单选_第76路"(w129) -> ()
              n4444 = local write "单选_第77路"(w129) -> ()
              n4445 = local write "单选_第78路"(w129) -> ()
              n4446 = local write "单选_第80路"(w129) -> ()
            }
            frame 51 {
              w130 = TRUE
              w131 = FALSE ("单选_第41路")
              n4447 = local write "单选_第1路"(w130) -> ()
              n4448 = local write "单选_第2路"(w130) -> ()
              n4449 = local write "单选_第3路"(w130) -> ()
              n4450 = local write "单选_第4路"(w130) -> ()
              n4451 = local write "单选_第5路"(w130) -> ()
              n4452 = local write "单选_第6路"(w130) -> ()
              n4453 = local write "单选_第7路"(w130) -> ()
              n4454 = local write "单选_第8路"(w130) -> ()
              n4455 = local write "单选_第9路"(w130) -> ()
              n4456 = local write "单选_第10路"(w130) -> ()
              n4457 = local write "单选_第11路"(w130) -> ()
              n4458 = local write "单选_第12路"(w130) -> ()
              n4459 = local write "单选_第13路"(w130) -> ()
              n4460 = local write "单选_第14路"(w130) -> ()
              n4461 = local write "单选_第15路"(w130) -> ()
              n4462 = local write "单选_第16路"(w130) -> ()
              n4463 = local write "单选_第17路"(w130) -> ()
              n4464 = local write "单选_第18路"(w130) -> ()
              n4465 = local write "单选_第19路"(w130) -> ()
              n4466 = local write "单选_第20路"(w130) -> ()
              n4467 = local write "单选_第21路"(w130) -> ()
              n4468 = local write "单选_第22路"(w130) -> ()
              n4469 = local write "单选_第23路"(w130) -> ()
              n4470 = local write "单选_第24路"(w130) -> ()
              n4471 = local write "单选_第25路"(w130) -> ()
              n4472 = local write "单选_第26路"(w130) -> ()
              n4473 = local write "单选_第27路"(w130) -> ()
              n4474 = local write "单选_第28路"(w130) -> ()
              n4475 = local write "单选_第29路"(w130) -> ()
              n4476 = local write "单选_第30路"(w130) -> ()
              n4477 = local write "单选_第31路"(w130) -> ()
              n4478 = local write "单选_第32路"(w130) -> ()
              n4479 = local write "单选_第33路"(w130) -> ()
              n4480 = local write "单选_第34路"(w130) -> ()
              n4481 = local write "单选_第35路"(w130) -> ()
              n4482 = local write "单选_第36路"(w130) -> ()
              n4483 = local write "单选_第37路"(w130) -> ()
              n4484 = local write "单选_第38路"(w130) -> ()
              n4485 = local write "单选_第39路"(w130) -> ()
              n4486 = local write "单选_第40路"(w130) -> ()
              n4487 = local write "单选_第41路"(w130) -> ()
              n4488 = local write "单选_第42路"(w130) -> ()
              n4489 = local write "单选_第43路"(w130) -> ()
              n4490 = local write "单选_第44路"(w130) -> ()
              n4491 = local write "单选_第45路"(w130) -> ()
              n4492 = local write "单选_第46路"(w130) -> ()
              n4493 = local write "单选_第47路"(w130) -> ()
              n4494 = local write "单选_第48路"(w130) -> ()
              n4495 = local write "单选_第49路"(w130) -> ()
              n4496 = local write "单选_第50路"(w130) -> ()
              n4497 = local write "单选_第51路"(w130) -> ()
              n4498 = local write "单选_第52路"(w131) -> ()
              n4499 = local write "单选_第53路"(w131) -> ()
              n4500 = local write "单选_第54路"(w131) -> ()
              n4501 = local write "单选_第55路"(w131) -> ()
              n4502 = local write "单选_第56路"(w131) -> ()
              n4503 = local write "单选_第57路"(w131) -> ()
              n4504 = local write "单选_第58路"(w131) -> ()
              n4505 = local write "单选_第59路"(w131) -> ()
              n4506 = local write "单选_第60路"(w131) -> ()
              n4507 = local write "单选_第61路"(w131) -> ()
              n4508 = local write "单选_第62路"(w131) -> ()
              n4509 = local write "单选_第63路"(w131) -> ()
              n4510 = local write "单选_第64路"(w131) -> ()
              n4511 = local write "单选_第71路"(w131) -> ()
              n4512 = local write "单选_第79路"(w131) -> ()
              n4513 = local write "单选_第65路"(w131) -> ()
              n4514 = local write "单选_第66路"(w131) -> ()
              n4515 = local write "单选_第67路"(w131) -> ()
              n4516 = local write "单选_第68路"(w131) -> ()
              n4517 = local write "单选_第69路"(w131) -> ()
              n4518 = local write "单选_第70路"(w131) -> ()
              n4519 = local write "单选_第72路"(w131) -> ()
              n4520 = local write "单选_第73路"(w131) -> ()
              n4521 = local write "单选_第74路"(w131) -> ()
              n4522 = local write "单选_第75路"(w131) -> ()
              n4523 = local write "单选_第76路"(w131) -> ()
              n4524 = local write "单选_第77路"(w131) -> ()
              n4525 = local write "单选_第78路"(w131) -> ()
              n4526 = local write "单选_第80路"(w131) -> ()
            }
            frame 52 {
              w132 = TRUE
              w133 = FALSE ("单选_第41路")
              n4527 = local write "单选_第1路"(w132) -> ()
              n4528 = local write "单选_第2路"(w132) -> ()
              n4529 = local write "单选_第3路"(w132) -> ()
              n4530 = local write "单选_第4路"(w132) -> ()
              n4531 = local write "单选_第5路"(w132) -> ()
              n4532 = local write "单选_第6路"(w132) -> ()
              n4533 = local write "单选_第7路"(w132) -> ()
              n4534 = local write "单选_第8路"(w132) -> ()
              n4535 = local write "单选_第9路"(w132) -> ()
              n4536 = local write "单选_第10路"(w132) -> ()
              n4537 = local write "单选_第11路"(w132) -> ()
              n4538 = local write "单选_第12路"(w132) -> ()
              n4539 = local write "单选_第13路"(w132) -> ()
              n4540 = local write "单选_第14路"(w132) -> ()
              n4541 = local write "单选_第15路"(w132) -> ()
              n4542 = local write "单选_第16路"(w132) -> ()
              n4543 = local write "单选_第17路"(w132) -> ()
              n4544 = local write "单选_第18路"(w132) -> ()
              n4545 = local write "单选_第19路"(w132) -> ()
              n4546 = local write "单选_第20路"(w132) -> ()
              n4547 = local write "单选_第21路"(w132) -> ()
              n4548 = local write "单选_第22路"(w132) -> ()
              n4549 = local write "单选_第23路"(w132) -> ()
              n4550 = local write "单选_第24路"(w132) -> ()
              n4551 = local write "单选_第25路"(w132) -> ()
              n4552 = local write "单选_第26路"(w132) -> ()
              n4553 = local write "单选_第27路"(w132) -> ()
